vi "Get value string.vi"(8 "error in (no error)":errorcluster, 11 "Column in":refnum<class "Text Field.lvclass">) -> (0 "error out":errorcluster, 2 "Value":string, 3 "Column out":refnum<class "Text Field.lvclass">)   [LabVIEW 2020]
uses:
  Text Field.lvclass
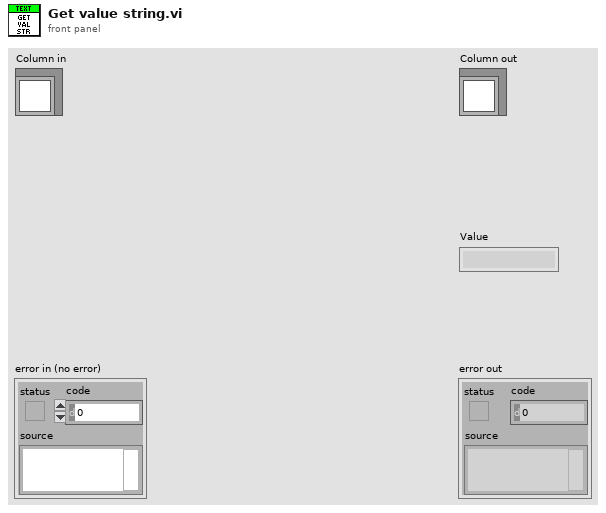
[diagram p1: front panel]
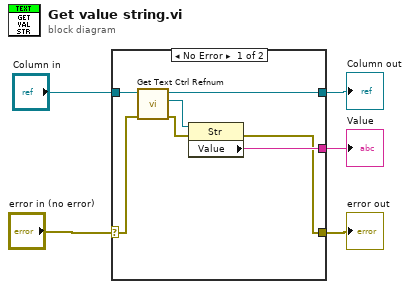
[diagram p0: block diagram]
diagram:
  n1 = case shown="No Error" "error in (no error)" {
    selector: "error in (no error)" -> [w10 w14]
    tunnel: "Column in" -> [w12 w13]
    tunnel: [w6 w14] -> w3
    tunnel: [w11 w13] -> w2
    tunnel: [w7 _] -> w1
    frame No Error {
      n2 = call "Get Text Ctrl Refnum.vi"("error in (no error)"=w10, "Text Field in"=w12) -> ("error out"=w8:errorcluster, "Text Refnum"=w9:refnum<vi>, "Text Field out"=w11:refnum<class "Text Field.lvclass">)  [unwired: 7 in]
      n3 = property class="Str"(reference=w9, error in=w8) -> (error out=w6:errorcluster, "Value"=w7:string)  [unwired: 1 out]
    }
    frame Error {
    }
  }
  "error out" <- w3
  "Column out" <- w2
  "Value" <- w1
